vi "Get Events.vi"(11 "CANopen Master in":refnum<class "CANopen Master.lvclass">) -> (2 "Events":T1, 3 "CANopen Master out":refnum<class "CANopen Master.lvclass">)   [LabVIEW 2024, in "CANopen Master.lvlib" / "CANopen Master.lvclass"]
uses:
  CANopen Master.lvclass
  CANopen Master.lvclass/CANopen Master.ctl
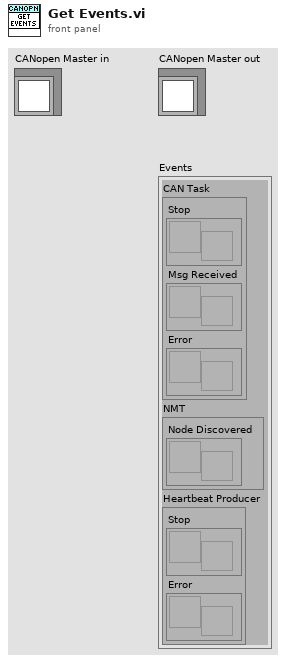
[diagram p1: front panel]
types:
  T1 = cluster{"CAN Task":cluster{"Stop":refnum<user-event>, "Msg Received":refnum<user-event>, "Error":refnum<user-event>}, "NMT":cluster{"Node Discovered":refnum<user-event>}, "Heartbeat Producer":cluster{"Stop":refnum<user-event>, "Error":refnum<user-event>}}
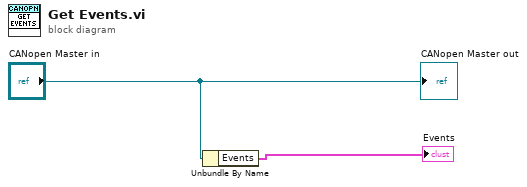
[diagram p0: block diagram]
diagram:
  n1 = Unbundle By Name("CANopen Master in") -> ("Events"=→"Events":T1)
  "CANopen Master out" <- "CANopen Master in"
